vi "Benchmark_SetName.vi"() -> ()   [LabVIEW 2013]
uses:
  source/Variant/OpenVariant.lvlib
panel:
  out "Waveform Chart":dbl(graph)
  out "execution time per call":dbl
  out "Array":variant[](array[variant])
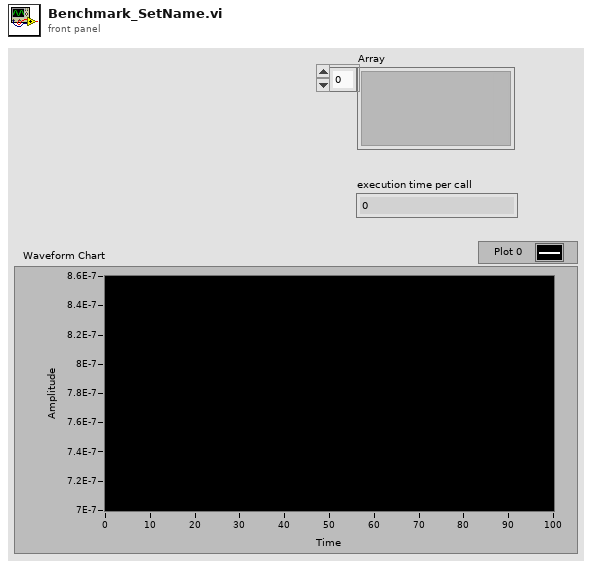
[diagram p1: front panel]
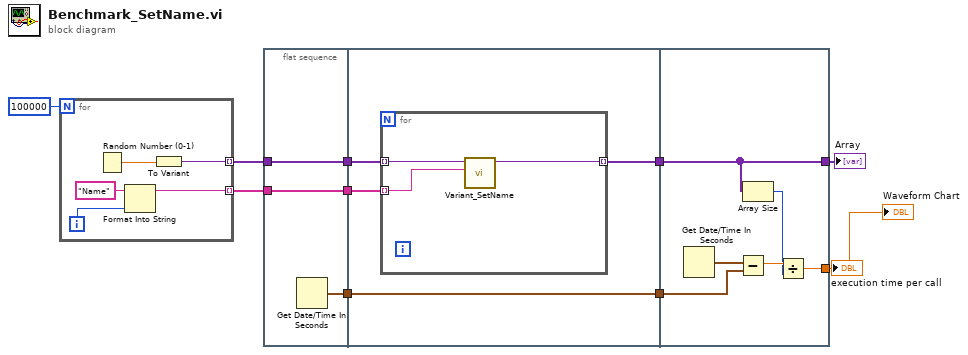
[diagram p0: block diagram]
diagram:
  n1 = for {
    N: 100000 -> [_]
    tunnel: [w14] -> w9 mode=indexing
    tunnel: [w11] -> w8 mode=indexing
    i -> [w13]
    n2 = Random Number (0-1)() -> (number: 0 to 1=w15:dbl)
    n3 = Format Into String(initial string="Name", w13) -> (resulting string=w11:string)  [unwired: 2 in, 1 out]
    n4 = To Variant(anything=w15) -> (Variant=w14:variant)
  }
  n5 = flat-sequence {
    tunnel: w8 -> [w17]
    tunnel: w9 -> [w18]
    tunnel: [w18] -> w5
    tunnel: [w17] -> w4
    tunnel: [w16] -> w2
    tunnel: [w20] -> w6
    tunnel: w5 -> [w22]
    tunnel: w4 -> [w21]
    tunnel: [w19] -> w3
    tunnel: w2 -> [w19]
    tunnel: [w28] -> w7
    tunnel: w6 -> [w28]
    tunnel: w3 -> [w30]
    tunnel: [w26] -> w1
    frame #0 {
      n6 = Get Date/Time In Seconds() -> (seconds since 1Jan1904=w16:timestamp)
    }
    frame #1 {
      n7 = for {
        tunnel: w22 -> [w25] mode=indexing
        tunnel: w21 -> [w23] mode=indexing
        tunnel: [w24] -> w20 mode=indexing
        n8 = call "Variant_SetName.vi"("Name"=w23, "Variant"=w25) -> ("Named Variant"=w24:variant)  [unwired: 9 in]
      }
    }
    frame #2 {
      n9 = Get Date/Time In Seconds() -> (seconds since 1Jan1904=w31:timestamp)
      n10 = Subtract(x=w31, y=w30) -> (x-y=w29:dbl)
      n11 = Array Size(array=w28) -> (size(s)=w27:i32)
      n12 = Divide(x=w29, y=w27) -> (x/y=w26:dbl)
    }
  }
  "Array" <- w7
  "execution time per call" <- w1
  "Waveform Chart" <- w1
